vi "Get Default Buffer.vi"(8 "error in (no error)":errorcluster, 11 "DMM6500 in":refnum<class "DMM6500.lvclass">) -> (0 "error out":errorcluster, 2 "Buffer":string="defBuffer1", 3 "DMM6500 out":refnum<class "DMM6500.lvclass">)   [LabVIEW 2023, in "HAF.lvlib" / "DMM6500.lvclass"]
doc: "Returns the name of the default Buffer. Subclasses should override if buffers are used by the interfaced Instrument and a default is specified in its programming manual. This will ensure that commands are syntactically correct.\n\nThe default is to return an empty String."
uses:
  DMM6500.lvclass
  DMM6500.lvclass/DMM6500.ctl
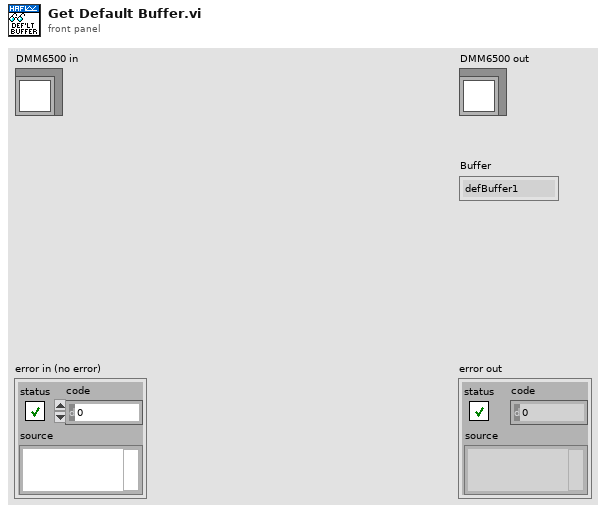
[diagram p1: front panel]
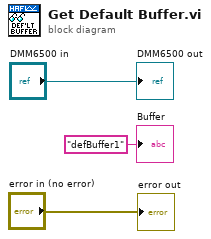
[diagram p0: block diagram]
diagram:
  "error out" <- "error in (no error)"
  "DMM6500 out" <- "DMM6500 in"
  "Buffer" <- "defBuffer1" ("Buffer")
